vi "Get_INI_UUT_Section.vi"(8 "error in (no error)":errorcluster, 9 "Sequence Path":path, 10 "Section Name":string="UUT", 11 "name or relative path":string="ModisEdge.ini") -> (0 "error out":errorcluster, 1 "PcbAssyNo":string, 2 "ManufactLocation":string, 3 "ManufactDate":string, 4 "LastCalLocation":string, 5 "PcbRev":string)   [LabVIEW 2015]
uses:
  <vilib>/Utility/config.llb/Read Key (String).vi
  <vilib>/Utility/config.llb/NI_LVConfig.lvlib
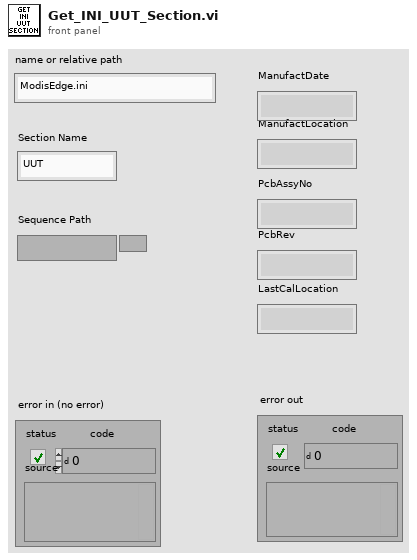
[diagram p1: front panel]
types:
  T1 = typedef "NI_LVConfig.lvlib/Config Data RefNum.ctl" = refnum<k1>
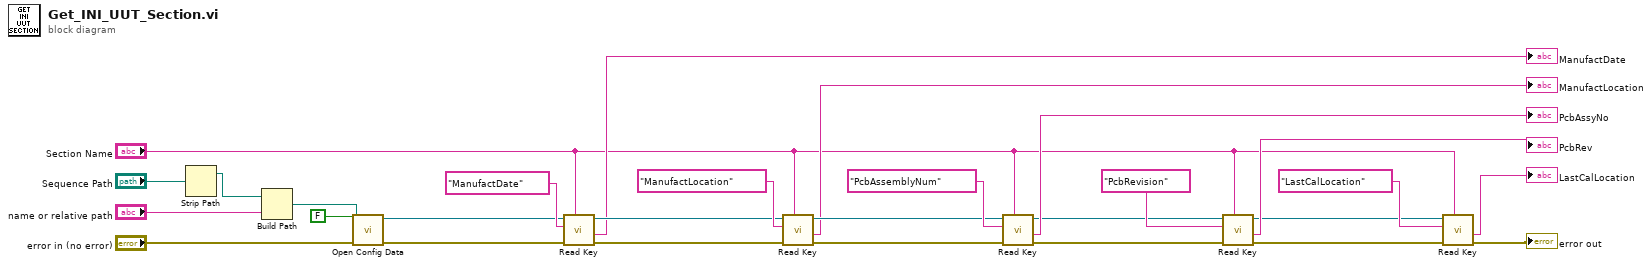
[diagram p0: block diagram]
diagram:
  n1 = Strip Path(path="Sequence Path") -> (stripped path=w2:path)  [unwired: 1 out]
  n2 = Build Path(base path=w2, name or relative path="name or relative path") -> (appended path=w8:path)
  n3 = call <vilib>:"Open Config Data.vi"("error in (no error)"="error in (no error)", "create file if necessary (T)"=FALSE, "configuration file path"=w8) -> ("error out"=w6:errorcluster, "refnum"=w5:T1)  [unwired: 6 in, 1 out]
  n4 = call-poly <vilib>:"Read Key.vi"("section"="Section Name", "error in (no error)"=w6, "key"="ManufactDate", "refnum"=w5) -> ("error out"=w17:errorcluster, "value"=→"ManufactDate":string, "refnum out"=w16:T1)  [unwired: 4 in, 1 out]
  n5 = call-poly <vilib>:"Read Key.vi"("section"="Section Name", "error in (no error)"=w17, "key"="ManufactLocation", "refnum"=w16) -> ("error out"=w20:errorcluster, "value"=→"ManufactLocation":string, "refnum out"=w21:T1)  [unwired: 4 in, 1 out]
  n6 = call-poly <vilib>:"Read Key.vi"("section"="Section Name", "error in (no error)"=w20, "key"="PcbAssemblyNum", "refnum"=w21) -> ("error out"=w25:errorcluster, "value"=→"PcbAssyNo":string, "refnum out"=w22:T1)  [unwired: 4 in, 1 out]
  n7 = call-poly <vilib>:"Read Key.vi"("section"="Section Name", "error in (no error)"=w25, "key"="PcbRevision", "refnum"=w22) -> ("error out"=w13:errorcluster, "value"=→"PcbRev":string, "refnum out"=w11:T1)  [unwired: 4 in, 1 out]
  n8 = call-poly <vilib>:"Read Key.vi"("section"="Section Name", "error in (no error)"=w13, "key"="LastCalLocation", "refnum"=w11) -> ("error out"=→"error out":errorcluster, "value"=→"LastCalLocation":string)  [unwired: 4 in, 2 out]
